vi "DIN Logic FPGA.vi"(0 "DIO Module":u8, 1 "Error Line Status":bool, 2 "Output Module Ready":bool, 5 "Masks":T1={"DIN1 Mask Out1"=[FALSE, FALSE, FALSE, FALSE, FALSE, FALSE, FALSE, FALSE], "DIN1 Mask Out2"=[FALSE, FALSE, FALSE, FALSE, FALSE, FALSE, FALSE, FALSE], "DIN1 Mask Out3"=[FALSE, FALSE, FALSE, FALSE, FALSE, FALSE, FALSE, FALSE], "DIN1 Mask Out4"=[FALSE, FALSE, FALSE, FALSE, FALSE, FALSE, FALSE, FALSE]}, 9 "External trigger":bool, 11 "Error":bool, 12 "ADC Triggered":bool, 13 "Interlock on":bool, 14 "Global Triggered":bool) -> (3 "Interlock Condition":cluster{bool, bool, bool, bool}, 6 "Global Triggered":bool, 8 "DIN Triggered Out":cluster{bool, bool, bool, bool}, 10 "DIN TrigMask Out":bool[](array[boolean]))   [LabVIEW 2014]
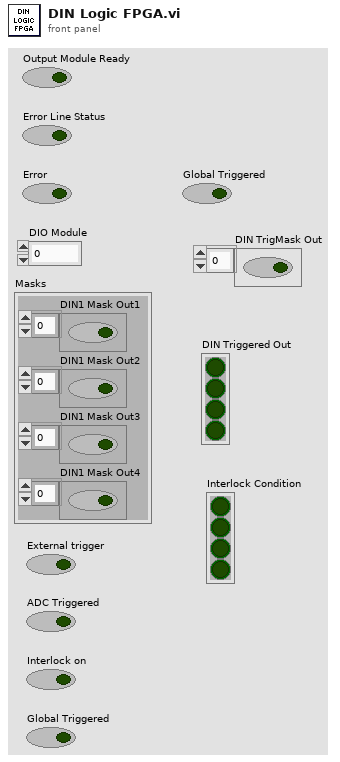
[diagram p1: front panel]
types:
  T1 = cluster{"DIN1 Mask Out1":bool[], "DIN1 Mask Out2":bool[], "DIN1 Mask Out3":bool[], "DIN1 Mask Out4":bool[]}
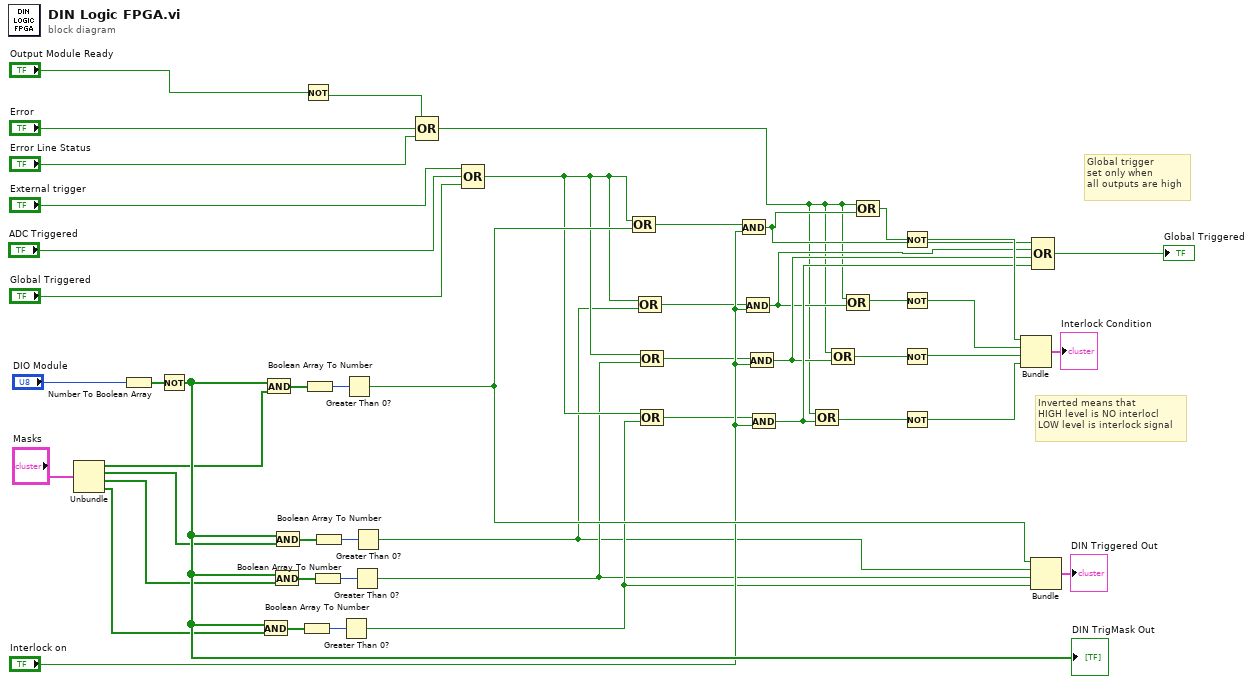
[diagram p0: block diagram]
diagram:
  # "Global trigger\nset only when \nall outputs are high"
  # "Inverted means that\nHIGH level is NO interlocl\nLOW level is interlock signal"
  n1 = Unbundle("Masks") -> ("DIN1 Mask Out1"=w32:bool[], "DIN1 Mask Out2"=w31:bool[], "DIN1 Mask Out3"=w30:bool[], "DIN1 Mask Out4"=w29:bool[])
  n2 = Number To Boolean Array(number="DIO Module") -> (Boolean array=w42:bool[])
  n3 = Not(x=w42) -> (.not. x?=w33:bool[])
  "DIN TrigMask Out" <- w33
  n4 = And(x=w33, y=w29) -> (x .and. y?=w35:bool[])
  n5 = And(x=w33, y=w32) -> (x .and. y?=w41:bool[])
  n6 = And(x=w33, y=w30) -> (x .and. y?=w37:bool[])
  n7 = And(x=w33, y=w31) -> (x .and. y?=w36:bool[])
  n8 = Boolean Array To Number(Boolean array=w35) -> (number=w34:u8)
  n9 = Not(x="Output Module Ready") -> (.not. x?=w49:bool)
  n10 = Boolean Array To Number(Boolean array=w41) -> (number=w43:u8)
  n11 = Boolean Array To Number(Boolean array=w37) -> (number=w38:u8)
  n12 = Boolean Array To Number(Boolean array=w36) -> (number=w39:u8)
  n13 = Greater Than 0?(x=w34) -> (x > 0?=w20:bool)
  n14 = Greater Than 0?(x=w43) -> (x > 0?=w28:bool)
  n15 = Greater Than 0?(x=w38) -> (x > 0?=w19:bool)
  n16 = Greater Than 0?(x=w39) -> (x > 0?=w18:bool)
  n17 = Compound Arithmetic op=OR(w49, "Error", "Error Line Status") -> (w2:bool)
  n18 = Compound Arithmetic op=OR("External trigger", "ADC Triggered", "Global Triggered") -> (w21:bool)
  n19 = Compound Arithmetic op=OR(w21, w28) -> (w46:bool)
  n20 = Compound Arithmetic op=OR(w21, w18) -> (w17:bool)
  n21 = Compound Arithmetic op=OR(w21, w19) -> (w16:bool)
  n22 = Compound Arithmetic op=OR(w21, w20) -> (w15:bool)
  n23 = And(x=w46, y="Interlock on") -> (x .and. y?=w6:bool)
  n24 = And(x=w17, y="Interlock on") -> (x .and. y?=w3:bool)
  n25 = And(x=w16, y="Interlock on") -> (x .and. y?=w4:bool)
  n26 = And(x=w15, y="Interlock on") -> (x .and. y?=w5:bool)
  n27 = Compound Arithmetic op=OR(w2, w5) -> (w12:bool)
  n28 = Compound Arithmetic op=OR(w2, w4) -> (w13:bool)
  n29 = Compound Arithmetic op=OR(w2, w3) -> (w14:bool)
  n30 = Compound Arithmetic op=OR(w2, w6) -> (w26:bool)
  n31 = Not(x=w26) -> (.not. x?=w9:bool)
  n32 = Not(x=w14) -> (.not. x?=w8:bool)
  n33 = Not(x=w13) -> (.not. x?=w10:bool)
  n34 = Not(x=w12) -> (.not. x?=w11:bool)
  n35 = Bundle(w9, w8, w10, w11) -> (→"Interlock Condition":cluster{bool, bool, bool, bool})  [unwired: 1 in]
  n36 = Bundle(w28, w18, w19, w20) -> (→"DIN Triggered Out":cluster{bool, bool, bool, bool})  [unwired: 1 in]
  n37 = Compound Arithmetic op=OR(w6, w3, w4, w5) -> (→"Global Triggered":bool)
